vi "App - analyze RUS V6.vi"() -> ()   [LabVIEW 2015] (continued)
"phase"=4.207063834838992, "Q"=7083.997208863392, "Norm  Ampl"=0.042629920830408, "z (inf)"=0.4164640226070026-0.2153386241198867i, "4corners"={"z (-pi/2)"=-0.19933862411988668-0.3924640226070026i, "z(inf)"=0.4164640226070026-0.2153386241198867i, "z (pi/2)"=0.2393386241198867+0.4004640226070026i, "z center"=0.020000000000000018+0.0040000000000000036i, "z(0)"=-0.37646402260700257+0.2233386241198867i, "radius"=0.4530928748640071}}, "timestamp(min)"=241.9666666686535, "timestamp"=timestamp(3493742339 s since 1904-01-01), "Magn Field(T)"=0.0}, {"temperature"=175.963, "lorentzian"={"Amplitude"=0.0005260699966110523, "omega(0)"=666.5273905158227, "Gamma"=0.09447421907192355, "phase"=4.195778497264702, "Q"=7055.124636789992, "Norm  Ampl"=0.042809672171456516, "z (inf)"=0.41400103807529176-0.21982010606648514i, "4corners"={"z (-pi/2)"=-0.20382010606648512-0.39000103807529174i, "z(inf)"=0.41400103807529176-0.21982010606648514i, "z (pi/2)"=0.24382010606648516+0.39800103807529175i, "z center"=0.020000000000000018+0.0040000000000000036i, "z(0)"=-0.3740010380752917+0.22782010606648515i, "radius"=0.45313602580684326}}, "timestamp(min)"=243.2833333313465, "timestamp"=timestamp(3493742418 s since 1904-01-01), "Magn Field(T)"=0.0}, {"temperature"=175.634, "lorentzian"={"Amplitude"=0.000521344887977522, "omega(0)"=666.5408565163474, "Gamma"=0.09513732241648067, "phase"=4.19366498389086, "Q"=7006.092242100796, "Norm  Ampl"=0.04303036973253523, "z (inf)"=0.4127988612141764-0.22823659659492584i, "4corners"={"z (-pi/2)"=-0.20423659659492582-0.3967988612141764i, "z(inf)"=0.4127988612141764-0.22823659659492584i, "z (pi/2)"=0.24423659659492586+0.3887988612141764i, "z center"=0.020000000000000018-0.0040000000000000036i, "z(0)"=-0.3727988612141764+0.22023659659492584i, "radius"=0.4522974647548108}}, "timestamp(min)"=244.60000000149012, "timestamp"=timestamp(3493742497 s since 1904-01-01), "Magn Field(T)"=0.0}, {"temperature"=175.302, "lorentzian"={"Amplitude"=0.0005173979173400528, "omega(0)"=666.5638551761065, "Gamma"=0.0938468907422214, "phase"=4.179539778200027, "Q"=7102.6738329245645, "Norm  Ampl"=0.04236278976880251, "z (inf)"=0.40882213382141586-0.2333081460968691i, "4corners"={"z (-pi/2)"=-0.20930814609686907-0.39282213382141584i, "z(inf)"=0.40882213382141586-0.2333081460968691i, "z (pi/2)"=0.2493081460968691+0.38482213382141583i, "z center"=0.020000000000000018-0.0040000000000000036i, "z(0)"=-0.3688221338214158+0.22530814609686908i, "radius"=0.4514032317294839}}, "timestamp(min)"=245.93333333730698, "timestamp"=timestamp(3493742577 s since 1904-01-01), "Magn Field(T)"=0.0}, {"temperature"=174.985, "lorentzian"={"Amplitude"=0.0005254947174563582, "omega(0)"=666.584524931986, "Gamma"=0.09467228615844603, "phase"=4.174992240459032, "Q"=7040.967869059089, "Norm  Ampl"=0.04284549568400563, "z (inf)"=0.40877454210818925-0.22766937952883107i, "4corners"={"z (-pi/2)"=-0.21166937952883105-0.38477454210818923i, "z(inf)"=0.40877454210818925-0.22766937952883107i, "z (pi/2)"=0.25166937952883106+0.39277454210818924i, "z center"=0.020000000000000018+0.0040000000000000036i, "z(0)"=-0.3687745421081892+0.23566937952883107i, "radius"=0.4525663995511662}}, "timestamp(min)"=247.25, "timestamp"=timestamp(3493742656 s since 1904-01-01), "Magn Field(T)"=0.0}, {"temperature"=174.654, "lorentzian"={"Amplitude"=0.0005181490056271822, "omega(0)"=666.5994517164672, "Gamma"=0.09372303123313948, "phase"=4.158300486836943, "Q"=7112.440164875554, "Norm  Ampl"=0.042653947239770486, "z (inf)"=0.40701352496332366-0.2354625794994841i, "4corners"={"z (-pi/2)"=-0.21946257949948408-0.38301352496332364i, "z(inf)"=0.40701352496332366-0.2354625794994841i, "z (pi/2)"=0.25946257949948415+0.39101352496332364i, "z center"=0.020000000000000018+0.0040000000000000036i, "z(0)"=-0.3670135249633236+0.2434625794994841i, "radius"=0.4551063562345442}}, "timestamp(min)"=248.5666666701436, "timestamp"=timestamp(3493742735 s since 1904-01-01), "Magn Field(T)"=0.0}, {"temperature"=174.316, "lorentzian"={"Amplitude"=0.0005205950851143368, "omega(0)"=666.6209744644639, "Gamma"=0.09378760365181929, "phase"=4.155628442977468, "Q"=7107.772760025443, "Norm  Ampl"=0.04260755617709387, "z (inf)"=0.4056863388300806-0.23606887328625673i, "4corners"={"z (-pi/2)"=-0.2200688732862567-0.3816863388300806i, "z(inf)"=0.4056863388300806-0.23606887328625673i, "z (pi/2)"=0.2600688732862567+0.3896863388300806i, "z center"=0.020000000000000018+0.0040000000000000036i, "z(0)"=-0.36568633883008056+0.24406887328625673i, "radius"=0.4542983775901962}}, "timestamp(min)"=249.89999999850988, "timestamp"=timestamp(3493742815 s since 1904-01-01), "Magn Field(T)"=0.0}, {"temperature"=173.984, "lorentzian"={"Amplitude"=0.0005205939429529912, "omega(0)"=666.6398754592545, "Gamma"=0.09417963894260288, "phase"=4.150745972928352, "Q"=7078.386400117052, "Norm  Ampl"=0.04256979081159615, "z (inf)"=0.4025696519710433-0.23672840118410748i, "4corners"={"z (-pi/2)"=-0.22072840118410747-0.37856965197104325i, "z(inf)"=0.4025696519710433-0.23672840118410748i, "z (pi/2)"=0.2607284011841075+0.38656965197104326i, "z center"=0.020000000000000018+0.0040000000000000036i, "z(0)"=-0.36256965197104324+0.2447284011841075i, "radius"=0.4520063071970365}}, "timestamp(min)"=251.2166666686535, "timestamp"=timestamp(3493742894 s since 1904-01-01), "Magn Field(T)"=0.0}, {"temperature"=173.642, "lorentzian"={"Amplitude"=0.0005241695908499409, "omega(0)"=666.6584173096262, "Gamma"=0.09555208085544614, "phase"=4.155181311724554, "Q"=6976.91155798235, "Norm  Ampl"=0.04284869920904903, "z (inf)"=0.40060074366188225-0.24113954351394265i, "4corners"={"z (-pi/2)"=-0.21713954351394263-0.38460074366188224i, "z(inf)"=0.40060074366188225-0.24113954351394265i, "z (pi/2)"=0.25713954351394264+0.37660074366188223i, "z center"=0.020000000000000018-0.0040000000000000036i, "z(0)"=-0.3606007436618822+0.23313954351394264i, "radius"=0.44843292605915874}}, "timestamp(min)"=252.5333333313465, "timestamp"=timestamp(3493742973 s since 1904-01-01), "Magn Field(T)"=0.0}, {"temperature"=173.314, "lorentzian"={"Amplitude"=0.0005150928762822398, "omega(0)"=666.6738278296584, "Gamma"=0.09412889843388439, "phase"=4.129734532080279, "Q"=7082.562729637449, "Norm  Ampl"=0.04289883674194833, "z (inf)"=0.40054990465830365-0.24677056194440344i, "4corners"={"z (-pi/2)"=-0.23077056194440343-0.3765499046583036i, "z(inf)"=0.40054990465830365-0.24677056194440344i, "z (pi/2)"=0.27077056194440347+0.38454990465830363i, "z center"=0.020000000000000018+0.0040000000000000036i, "z(0)"=-0.3605499046583036+0.25477056194440345i, "radius"=0.45574565787657906}}, "timestamp(min)"=253.86666666716337, "timestamp"=timestamp(3493743053 s since 1904-01-01), "Magn Field(T)"=0.0}, {"temperature"=172.974, "lorentzian"={"Amplitude"=0.000516799692195644, "omega(0)"=666.692959166971, "Gamma"=0.09447287477688024, "phase"=4.135429912242744, "Q"=7056.977579453596, "Norm  Ampl"=0.042827204817983404, "z (inf)"=0.39994570670003854-0.24328038289100967i, "4corners"={"z (-pi/2)"=-0.22728038289100966-0.3759457067000385i, "z(inf)"=0.39994570670003854-0.24328038289100967i, "z (pi/2)"=0.2672803828910097+0.3839457067000385i, "z center"=0.020000000000000018+0.0040000000000000036i, "z(0)"=-0.3599457067000385+0.2512803828910097i, "radius"=0.4533280575946254}}, "timestamp(min)"=255.18333333730698, "timestamp"=timestamp(3493743132 s since 1904-01-01), "Magn Field(T)"=0.0}, {"temperature"=172.632, "lorentzian"={"Amplitude"=0.0005164262361548908, "omega(0)"=666.7084573649482, "Gamma"=0.09525334912451694, "phase"=4.119362082283542, "Q"=6999.3177509529305, "Norm  Ampl"=0.04303615866166019, "z (inf)"=0.3946624823159162-0.24850319278065613i, "4corners"={"z (-pi/2)"=-0.23250319278065612-0.3706624823159162i, "z(inf)"=0.3946624823159162-0.24850319278065613i, "z (pi/2)"=0.27250319278065616+0.3786624823159162i, "z center"=0.020000000000000018+0.0040000000000000036i, "z(0)"=-0.3546624823159162+0.25650319278065614i, "radius"=0.45180730186612683}}, "timestamp(min)"=256.5, "timestamp"=timestamp(3493743211 s since 1904-01-01), "Magn Field(T)"=0.0}, {"temperature"=172.303, "lorentzian"={"Amplitude"=0.0005144419777848418, "omega(0)"=666.7295180919369, "Gamma"=0.09498586850167676, "phase"=4.11250549518927, "Q"=7019.249585322972, "Norm  Ampl"=0.04256383601987101, "z (inf)"=0.3898681744046229-0.24897717189284335i, "4corners"={"z (-pi/2)"=-0.23297717189284334-0.3658681744046229i, "z(inf)"=0.3898681744046229-0.24897717189284335i, "z (pi/2)"=0.2729771718928434+0.3738681744046229i, "z center"=0.020000000000000018+0.0040000000000000036i, "z(0)"=-0.34986817440462287+0.25697717189284336i, "radius"=0.44810703624949894}}, "timestamp(min)"=257.83333333581686, "timestamp"=timestamp(3493743291 s since 1904-01-01), "Magn Field(T)"=0.0}, {"temperature"=171.947, "lorentzian"={"Amplitude"=0.0005056516743748706, "omega(0)"=666.7478022514588, "Gamma"=0.09481296917232077, "phase"=4.084832371198923, "Q"=7032.242614822634, "Norm  Ampl"=0.0422584021142444, "z (inf)"=0.38878060950325605-0.24970269914437565i, "4corners"={"z (-pi/2)"=-0.23370269914437564-0.348780609503256i, "z(inf)"=0.38878060950325605-0.24970269914437565i, "z (pi/2)"=0.2897026991443757+0.37278060950325603i, "z center"=0.028000000000000025+0.01200000000000001i, "z(0)"=-0.332780609503256+0.27370269914437567i, "radius"=0.44570276074194615}}, "timestamp(min)"=259.1499999985099, "timestamp"=timestamp(3493743370 s since 1904-01-01), "Magn Field(T)"=0.0}, {"temperature"=171.593, "lorentzian"={"Amplitude"=0.0004999937810113293, "omega(0)"=666.7684075589387, "Gamma"=0.07716584127533078, "phase"=4.101848615846865, "Q"=8640.71973478372, "Norm  Ampl"=0.04197129217223431, "z (inf)"=0.37764652347352495-0.2678293416658969i, "4corners"={"z (-pi/2)"=-0.37982934166589694-0.4016465234735249i, "z(inf)"=0.37764652347352495-0.2678293416658969i, "z (pi/2)"=0.24382934166589693+0.489646523473525i, "z center"=-0.068+0.04400000000000004i, "z(0)"=-0.513646523473525+0.35582934166589697i, "radius"=0.5439102519789691}}, "timestamp(min)"=260.4666666686535, "timestamp"=timestamp(3493743449 s since 1904-01-01), "Magn Field(T)"=0.0}, {"temperature"=171.216, "lorentzian"={"Amplitude"=0.0004971178519728986, "omega(0)"=666.7892001669214, "Gamma"=0.07709429273268266, "phase"=4.122089168704795, "Q"=8649.008591063302, "Norm  Ampl"=0.04142514157990056, "z (inf)"=0.37840040980273176-0.26308378893787776i, "4corners"={"z (-pi/2)"=-0.3670837889378778-0.41040040980273174i, "z(inf)"=0.37840040980273176-0.26308378893787776i, "z (pi/2)"=0.2310837889378778+0.4824004098027318i, "z center"=-0.068+0.03600000000000003i, "z(0)"=-0.5144004098027317+0.3350837889378778i, "radius"=0.5373308465717224}}, "timestamp(min)"=261.80000000447035, "timestamp"=timestamp(3493743529 s since 1904-01-01), "Magn Field(T)"=0.0}, {"temperature"=170.839, "lorentzian"={"Amplitude"=0.0005456618128673867, "omega(0)"=666.8168017277993, "Gamma"=0.10284084968364095, "phase"=4.2580332816999835, "Q"=6483.9682264300745, "Norm  Ampl"=0.0455123865470925, "z (inf)"=0.4016521142220204-0.26222859964929973i, "4corners"={"z (-pi/2)"=-0.19022859964929972-0.4656521142220204i, "z(inf)"=0.4016521142220204-0.26222859964929973i, "z (pi/2)"=0.19822859964929973+0.3296521142220204i, "z center"=0.0040000000000000036-0.068i, "z(0)"=-0.3936521142220204+0.12622859964929972i, "radius"=0.4425516386445436}}, "timestamp(min)"=263.1166666671634, "timestamp"=timestamp(3493743608 s since 1904-01-01), "Magn Field(T)"=0.0}, {"temperature"=170.496, "lorentzian"={"Amplitude"=0.0005526211872780759, "omega(0)"=666.8378173116613, "Gamma"=0.1050772709506424, "phase"=4.262296084777731, "Q"=6346.166124022129, "Norm  Ampl"=0.04629332333343278, "z (inf)"=0.40068729260806996-0.26766725748477393i, "4corners"={"z (-pi/2)"=-0.18766725748477392-0.47268729260806996i, "z(inf)"=0.40068729260806996-0.26766725748477393i, "z (pi/2)"=0.19566725748477393+0.32068729260806994i, "z center"=0.0040000000000000036-0.07600000000000001i, "z(0)"=-0.39268729260806995+0.11566725748477391i, "radius"=0.44056457609351113}}, "timestamp(min)"=264.45000000298023, "timestamp"=timestamp(3493743688 s since 1904-01-01), "Magn Field(T)"=0.0}, {"temperature"=170.187, "lorentzian"={"Amplitude"=0.0005512178829958511, "omega(0)"=666.8546119137043, "Gamma"=0.1059345471746253, "phase"=4.253770018900702, "Q"=6294.968258224992, "Norm  Ampl"=0.04649210092161766, "z (inf)"=0.40552439092601306-0.27029475928406893i, "4corners"={"z (-pi/2)"=-0.1822947592840689-0.46952439092601306i, "z(inf)"=0.40552439092601306-0.27029475928406893i, "z (pi/2)"=0.20629475928406893+0.31752439092601303i, "z center"=0.01200000000000001-0.07600000000000001i, "z(0)"=-0.38152439092601304+0.1182947592840689i, "radius"=0.43887572243055756}}, "timestamp(min)"=265.76666666567326, "timestamp"=timestamp(3493743767 s since 1904-01-01), "Magn Field(T)"=0.0}, {"temperature"=169.921, "lorentzian"={"Amplitude"=0.0004534509670476978, "omega(0)"=666.8518486216516, "Gamma"=0.07873324505819844, "phase"=3.841128173882247, "Q"=8469.762018937803, "Norm  Ampl"=0.03687627973060844, "z (inf)"=0.3295657315836148-0.3543691454307535i, "4corners"={"z (-pi/2)"=-0.33036914543075346-0.29756573158361477i, "z(inf)"=0.3295657315836148-0.3543691454307535i, "z (pi/2)"=0.3863691454307535+0.3055657315836148i, "z center"=0.028000000000000025+0.0040000000000000036i, "z(0)"=-0.27356573158361475+0.3623691454307535i, "radius"=0.46836986972085354}}, "timestamp(min)"=267.08333333581686, "timestamp"=timestamp(3493743846 s since 1904-01-01), "Magn Field(T)"=0.0}, {"temperature"=169.62, "lorentzian"={"Amplitude"=0.0004577554109132157, "omega(0)"=666.8670899449811, "Gamma"=0.07921421145205408, "phase"=3.886971896135157, "Q"=8418.52841454611, "Norm  Ampl"=0.037144170714167916, "z (inf)"=0.34603704562405213-0.340567947100091i, "4corners"={"z (-pi/2)"=-0.31656794710009095-0.3140370456240521i, "z(inf)"=0.34603704562405213-0.340567947100091i, "z (pi/2)"=0.372567947100091+0.3220370456240521i, "z center"=0.028000000000000025+0.0040000000000000036i, "z(0)"=-0.2900370456240521+0.348567947100091i, "radius"=0.4689079147956947}}, "timestamp(min)"=268.41666666418314, "timestamp"=timestamp(3493743926 s since 1904-01-01), "Magn Field(T)"=0.0}, {"temperature"=169.281, "lorentzian"={"Amplitude"=0.00046944630009999427, "omega(0)"=666.8864924413293, "Gamma"=0.08140026041873821, "phase"=3.8927509584525866, "Q"=8192.682541932176, "Norm  Ampl"=0.03810852720739882, "z (inf)"=0.3555140821106168-0.33817922533891204i, "4corners"={"z (-pi/2)"=-0.306179225338912-0.31551408211061677i, "z(inf)"=0.3555140821106168-0.33817922533891204i, "z (pi/2)"=0.3781792253389121+0.3235140821106168i, "z center"=0.03600000000000003+0.0040000000000000036i, "z(0)"=-0.28351408211061674+0.34617922533891204i, "radius"=0.46816222713983224}}, "timestamp(min)"=269.73333333432674, "timestamp"=timestamp(3493744005 s since 1904-01-01), "Magn Field(T)"=0.0}, {"temperature"=168.934, "lorentzian"={"Amplitude"=0.0004819119123264662, "omega(0)"=666.9049225640731, "Gamma"=0.08428016108055618, "phase"=3.9625507106763167, "Q"=7912.952633379947, "Norm  Ampl"=0.03935184782972083, "z (inf)"=0.3776895090479562-0.3142135310893408i, "4corners"={"z (-pi/2)"=-0.2822135310893408-0.33768950904795614i, "z(inf)"=0.3776895090479562-0.3142135310893408i, "z (pi/2)"=0.35421353108934084+0.34568950904795614i, "z center"=0.03600000000000003+0.0040000000000000036i, "z(0)"=-0.3056895090479561+0.3222135310893408i, "radius"=0.46691709324223735}}, "timestamp(min)"=271.05000000447035, "timestamp"=timestamp(3493744084 s since 1904-01-01), "Magn Field(T)"=0.0}, {"temperature"=168.567, "lorentzian"={"Amplitude"=0.00047042517655521463, "omega(0)"=666.9154225888688, "Gamma"=0.08165669931390285, "phase"=3.811505793800036, "Q"=8167.308110570664, "Norm  Ampl"=0.03849323915197239, "z (inf)"=0.32070276046478424-0.36552156103182776i, "4corners"={"z (-pi/2)"=-0.34152156103182774-0.2887027604647842i, "z(inf)"=0.32070276046478424-0.36552156103182776i, "z (pi/2)"=0.3975215610318278+0.2967027604647842i, "z center"=0.028000000000000025+0.0040000000000000036i, "z(0)"=-0.2647027604647842+0.37352156103182776i, "radius"=0.47140331994068907}}, "timestamp(min)"=272.3833333328366, "timestamp"=timestamp(3493744164 s since 1904-01-01), "Magn Field(T)"=0.0}, {"temperature"=168.198, "lorentzian"={"Amplitude"=0.0004781228250890849, "omega(0)"=666.9360592058572, "Gamma"=0.08225432815562943, "phase"=3.827463656766192, "Q"=8108.218426439273, "Norm  Ampl"=0.03910988481638956, "z (inf)"=0.3371408667391544-0.36395481797701695i, "4corners"={"z (-pi/2)"=-0.3319548179770169-0.29714086673915435i, "z(inf)"=0.3371408667391544-0.36395481797701695i, "z (pi/2)"=0.403954817977017+0.30514086673915436i, "z center"=0.03600000000000003+0.0040000000000000036i, "z(0)"=-0.2651408667391543+0.37195481797701696i, "radius"=0.4754750989199211}}, "timestamp(min)"=273.70000000298023, "timestamp"=timestamp(3493744243 s since 1904-01-01), "Magn Field(T)"=0.0}, {"temperature"=166.235, "lorentzian"={"Amplitude"=0.00047412858472916974, "omega(0)"=666.9893085918818, "Gamma"=0.08335043874440105, "phase"=3.9520200721143324, "Q"=8002.229126078666, "Norm  Ampl"=0.03905346852303167, "z (inf)"=0.37549950878743527-0.3189162721305466i, "4corners"={"z (-pi/2)"=-0.28691627213054655-0.33549950878743523i, "z(inf)"=0.37549950878743527-0.3189162721305466i, "z (pi/2)"=0.3589162721305466+0.34349950878743524i, "z center"=0.03600000000000003+0.0040000000000000036i, "z(0)"=-0.3034995087874352+0.3269162721305466i, "radius"=0.46854544632682005}}, "timestamp(min)"=275.01666666567326, "timestamp"=timestamp(3493744322 s since 1904-01-01), "Magn Field(T)"=0.0}, {"temperature"=167.465, "lorentzian"={"Amplitude"=0.00046785835178995565, "omega(0)"=667.023179450894, "Gamma"=0.08370886544636703, "phase"=4.015493047204771, "Q"=7968.3696092890095, "Norm  Ampl"=0.03886231878697336, "z (inf)"=0.39200901049802483-0.2939781015424444i, "4corners"={"z (-pi/2)"=-0.2619781015424444-0.3520090104980248i, "z(inf)"=0.39200901049802483-0.2939781015424444i, "z (pi/2)"=0.33397810154244445+0.3600090104980248i, "z center"=0.03600000000000003+0.0040000000000000036i, "z(0)"=-0.32000901049802477+0.3019781015424444i, "radius"=0.4642557103091162}}, "timestamp(min)"=276.3500000014901, "timestamp"=timestamp(3493744402 s since 1904-01-01), "Magn Field(T)"=0.0}, {"temperature"=167.68, "lorentzian"={"Amplitude"=0.0004660283199917108, "omega(0)"=667.0181290997397, "Gamma"=0.08122368655390495, "phase"=3.7880903220953956, "Q"=8212.11345359295, "Norm  Ampl"=0.03848331962891363, "z (inf)"=0.32141110368516546-0.37418188694120114i, "4corners"={"z (-pi/2)"=-0.3421818869412011-0.2814111036851654i, "z(inf)"=0.32141110368516546-0.37418188694120114i, "z (pi/2)"=0.41418188694120117+0.2894111036851654i, "z center"=0.03600000000000003+0.0040000000000000036i, "z(0)"=-0.2494111036851654+0.38218188694120114i, "radius"=0.4737942989496514}}, "timestamp(min)"=277.66666666418314, "timestamp"=timestamp(3493744481 s since 1904-01-01), "Magn Field(T)"=0.0}, {"temperature"=166.454, "lorentzian"={"Amplitude"=0.0004566778114597476, "omega(0)"=667.0522165263105, "Gamma"=0.07892871012914685, "phase"=3.8054289698611607, "Q"=8451.32544843123, "Norm  Ampl"=0.037899071353994104, "z (inf)"=0.33185238645268195-0.3741970972536763i, "4corners"={"z (-pi/2)"=-0.34219709725367625-0.2918523864526819i, "z(inf)"=0.33185238645268195-0.3741970972536763i, "z (pi/2)"=0.4141970972536763+0.2998523864526819i, "z center"=0.03600000000000003+0.0040000000000000036i, "z(0)"=-0.2598523864526819+0.3821970972536763i, "radius"=0.48016838602812423}}, "timestamp(min)"=279.0, "timestamp"=timestamp(3493744561 s since 1904-01-01), "Magn Field(T)"=0.0}, {"temperature"=166.595, "lorentzian"={"Amplitude"=0.0004415693097046763, "omega(0)"=667.0670953246381, "Gamma"=0.07763656776163326, "phase"=3.7695376107360197, "Q"=8592.176529141876, "Norm  Ampl"=0.036969393864618304, "z (inf)"=0.31575077270099183-0.3813465507477374i, "4corners"={"z (-pi/2)"=-0.34934655074773735-0.2757507727009918i, "z(inf)"=0.31575077270099183-0.3813465507477374i, "z (pi/2)"=0.4213465507477374+0.2837507727009918i, "z center"=0.03600000000000003+0.0040000000000000036i, "z(0)"=-0.24375077270099177+0.3893465507477374i, "radius"=0.47618532001730224}}, "timestamp(min)"=280.3166666701436, "timestamp"=timestamp(3493744640 s since 1904-01-01), "Magn Field(T)"=0.0}, {"temperature"=166.194, "lorentzian"={"Amplitude"=0.0004410364115785352, "omega(0)"=667.0830991408355, "Gamma"=0.07798823890009401, "phase"=3.736057416827716, "Q"=8553.637170796934, "Norm  Ampl"=0.03678081551395129, "z (inf)"=0.3001380691745166-0.37871285163862145i, "4corners"={"z (-pi/2)"=-0.35471285163862143-0.25213806917451653i, "z(inf)"=0.3001380691745166-0.37871285163862145i, "z (pi/2)"=0.4267128516386215+0.27613806917451655i, "z center"=0.03600000000000003+0.01200000000000001i, "z(0)"=-0.2281380691745165+0.40271285163862147i, "radius"=0.4716200292850433}}, "timestamp(min)"=281.6333333328366, "timestamp"=timestamp(3493744719 s since 1904-01-01), "Magn Field(T)"=0.0}, {"temperature"=165.738, "lorentzian"={"Amplitude"=0.0005310970253922922, "omega(0)"=667.0958987277553, "Gamma"=0.09231982716144078, "phase"=3.629992242151525, "Q"=7225.92230985438, "Norm  Ampl"=0.0441283586693555, "z (inf)"=0.3322812686918484-0.4421096316191092i, "4corners"={"z (-pi/2)"=-0.3141096316191092-0.2442812686918484i, "z(inf)"=0.3322812686918484-0.4421096316191092i, "z (pi/2)"=0.5301096316191092+0.20428126869184837i, "z center"=0.10799999999999998-0.020000000000000018i, "z(0)"=-0.1162812686918484+0.4021096316191092i, "radius"=0.4779943813389914}}, "timestamp(min)"=282.9666666686535, "timestamp"=timestamp(3493744799 s since 1904-01-01), "Magn Field(T)"=0.0}, {"temperature"=165.506, "lorentzian"={"Amplitude"=0.0004453500100210904, "omega(0)"=667.1178151875246, "Gamma"=0.07879774106191258, "phase"=3.724253916429, "Q"=8466.204820051376, "Norm  Ampl"=0.03683544160772606, "z (inf)"=0.29322348499012246-0.386336569477198i, "4corners"={"z (-pi/2)"=-0.354336569477198-0.2532234849901224i, "z(inf)"=0.29322348499012246-0.386336569477198i, "z (pi/2)"=0.42633656947719806+0.26122348499012243i, "z center"=0.03600000000000003+0.0040000000000000036i, "z(0)"=-0.2212234849901224+0.39433656947719803i, "radius"=0.46746824352215754}}, "timestamp(min)"=284.2833333313465, "timestamp"=timestamp(3493744878 s since 1904-01-01), "Magn Field(T)"=0.0}, {"temperature"=165.119, "lorentzian"={"Amplitude"=0.0005157776397258885, "omega(0)"=667.1376282461717, "Gamma"=0.09116435635561218, "phase"=3.709814210705731, "Q"=7317.965649247981, "Norm  Ampl"=0.04244970024471032, "z (inf)"=0.3585762630295389-0.41246837363300054i, "4corners"={"z (-pi/2)"=-0.28446837363300054-0.2705762630295389i, "z(inf)"=0.3585762630295389-0.41246837363300054i, "z (pi/2)"=0.5004683736330005+0.23057626302953887i, "z center"=0.10799999999999998-0.020000000000000018i, "z(0)"=-0.1425762630295389+0.3724683736330005i, "radius"=0.46563922504013894}}, "timestamp(min)"=285.6000000014901, "timestamp"=timestamp(3493744957 s since 1904-01-01), "Magn Field(T)"=0.0}, {"temperature"=164.781, "lorentzian"={"Amplitude"=0.0004418438472308204, "omega(0)"=667.1555761001051, "Gamma"=0.07827432143846805, "phase"=3.7454834472622567, "Q"=8523.300666675987, "Norm  Ampl"=0.03688829185154937, "z (inf)"=0.30361004228281907-0.3839171365651249i, "4corners"={"z (-pi/2)"=-0.35191713656512486-0.26361004228281903i, "z(inf)"=0.30361004228281907-0.3839171365651249i, "z (pi/2)"=0.4239171365651249+0.27161004228281904i, "z center"=0.03600000000000003+0.0040000000000000036i, "z(0)"=-0.231610042282819+0.3919171365651249i, "radius"=0.4712693917193201}}, "timestamp(min)"=286.933333337307, "timestamp"=timestamp(3493745037 s since 1904-01-01), "Magn Field(T)"=0.0}, {"temperature"=164.449, "lorentzian"={"Amplitude"=0.00043959014352216384, "omega(0)"=667.1729816030107, "Gamma"=0.07792122289310302, "phase"=3.7572404166451623, "Q"=8562.147215249412, "Norm  Ampl"=0.03705674417312184, "z (inf)"=0.31063385325452725-0.3842524925874322i, "4corners"={"z (-pi/2)"=-0.3522524925874322-0.2706338532545272i, "z(inf)"=0.31063385325452725-0.3842524925874322i, "z (pi/2)"=0.42425249258743225+0.2786338532545272i, "z center"=0.03600000000000003+0.0040000000000000036i, "z(0)"=-0.23863385325452718+0.3922524925874322i, "radius"=0.4755667685549352}}, "timestamp(min)"=288.25, "timestamp"=timestamp(3493745116 s since 1904-01-01), "Magn Field(T)"=0.0}, {"temperature"=164.092, "lorentzian"={"Amplitude"=0.00044484134846526204, "omega(0)"=667.1877067469779, "Gamma"=0.07911173500148858, "phase"=3.73486561224118, "Q"=8433.485964306357, "Norm  Ampl"=0.037600025703834174, "z (inf)"=0.3017170249130602-0.382059819707589i, "4corners"={"z (-pi/2)"=-0.358059819707589-0.25371702491306014i, "z(inf)"=0.3017170249130602-0.382059819707589i, "z (pi/2)"=0.43005981970758905+0.27771702491306016i, "z center"=0.03600000000000003+0.01200000000000001i, "z(0)"=-0.22971702491306012+0.40605981970758903i, "radius"=0.4752774756251609}}, "timestamp(min)"=289.58333333581686, "timestamp"=timestamp(3493745196 s since 1904-01-01), "Magn Field(T)"=0.0}, {"temperature"=163.762, "lorentzian"={"Amplitude"=0.00042567935379481, "omega(0)"=667.2026820856647, "Gamma"=0.07477989988062614, "phase"=3.664321115162137, "Q"=8922.219515548222, "Norm  Ampl"=0.035311410368920784, "z (inf)"=0.27174628774594833-0.40514648048645424i, "4corners"={"z (-pi/2)"=-0.3731464804864542-0.23174628774594827i, "z(inf)"=0.27174628774594833-0.40514648048645424i, "z (pi/2)"=0.4451464804864543+0.23974628774594828i, "z center"=0.03600000000000003+0.0040000000000000036i, "z(0)"=-0.19974628774594824+0.41314648048645425i, "radius"=0.47220456867807614}}, "timestamp(min)"=290.8999999985099, "timestamp"=timestamp(3493745275 s since 1904-01-01), "Magn Field(T)"=0.0}, {"temperature"=163.413, "lorentzian"={"Amplitude"=0.00041595713785414265, "omega(0)"=667.2204079387552, "Gamma"=0.07270858758415784, "phase"=3.6652170850341648, "Q"=9176.638277651442, "Norm  Ampl"=0.0343363115045469, "z (inf)"=0.2641332990001735-0.40497063950565165i, "4corners"={"z (-pi/2)"=-0.38097063950565163-0.2321332990001735i, "z(inf)"=0.2641332990001735-0.40497063950565165i, "z (pi/2)"=0.4369706395056517+0.2401332990001735i, "z center"=0.028000000000000025+0.0040000000000000036i, "z(0)"=-0.20813329900017347+0.41297063950565166i, "radius"=0.47224561286937017}}, "timestamp(min)"=292.2166666686535, "timestamp"=timestamp(3493745354 s since 1904-01-01), "Magn Field(T)"=0.0}, {"temperature"=163.066, "lorentzian"={"Amplitude"=0.000412780965095534, "omega(0)"=667.2371268200717, "Gamma"=0.072148551218395, "phase"=3.6596651214491858, "Q"=9248.101528751875, "Norm  Ampl"=0.03428932453282723, "z (inf)"=0.26335185326350824-0.40089420742790194i, "4corners"={"z (-pi/2)"=-0.3848942074279019-0.2233518532635082i, "z(inf)"=0.26335185326350824-0.40089420742790194i, "z (pi/2)"=0.440894207427902+0.24735185326350823i, "z center"=0.028000000000000025+0.01200000000000001i, "z(0)"=-0.2073518532635082+0.42489420742790196i, "radius"=0.47526005656070364}}, "timestamp(min)"=293.55000000447035, "timestamp"=timestamp(3493745434 s since 1904-01-01), "Magn Field(T)"=0.0}, {"temperature"=162.731, "lorentzian"={"Amplitude"=0.0004102842033046791, "omega(0)"=667.2364415496808, "Gamma"=0.07209084985268063, "phase"=3.6064865792014325, "Q"=9255.4941842577, "Norm  Ampl"=0.033756126499018595, "z (inf)"=0.24592700578322318-0.4145490860197161i, "4corners"={"z (-pi/2)"=-0.38254908601971604-0.20592700578322315i, "z(inf)"=0.24592700578322318-0.4145490860197161i, "z (pi/2)"=0.4545490860197161+0.21392700578322316i, "z center"=0.03600000000000003+0.0040000000000000036i, "z(0)"=-0.17392700578322312+0.4225490860197161i, "radius"=0.46824425801610114}}, "timestamp(min)"=294.8666666671634, "timestamp"=timestamp(3493745513 s since 1904-01-01), "Magn Field(T)"=0.0}, {"temperature"=162.385, "lorentzian"={"Amplitude"=0.0003956527969362258, "omega(0)"=667.2762898680271, "Gamma"=0.06962769430773084, "phase"=3.717337149894252, "Q"=9583.48968039774, "Norm  Ampl"=0.03259572680926661, "z (inf)"=0.29088493539914-0.3806724598159571i, "4corners"={"z (-pi/2)"=-0.3566724598159571-0.24288493539913997i, "z(inf)"=0.29088493539914-0.3806724598159571i, "z (pi/2)"=0.42867245981595714+0.26688493539914i, "z center"=0.03600000000000003+0.01200000000000001i, "z(0)"=-0.21888493539913995+0.4046724598159571i, "radius"=0.4681431308812917}}, "timestamp(min)"=296.20000000298023, "timestamp"=timestamp(3493745593 s since 1904-01-01), "Magn Field(T)"=0.0}, {"temperature"=162.052, "lorentzian"={"Amplitude"=0.0003908194038920824, "omega(0)"=667.2972094216088, "Gamma"=0.060554526875683225, "phase"=3.818969248519727, "Q"=11019.774141602189, "Norm  Ampl"=0.032463602340691455, "z (inf)"=0.2840045144273522-0.3737437622419629i, "4corners"={"z (-pi/2)"=-0.4697437622419629-0.29200451442735215i, "z(inf)"=0.2840045144273522-0.3737437622419629i, "z (pi/2)"=0.3657437622419629+0.3800045144273522i, "z center"=-0.05199999999999999+0.04400000000000004i, "z(0)"=-0.3880045144273522+0.46174376224196295i, "radius"=0.5361052924637383}}, "timestamp(min)"=297.51666666567326, "timestamp"=timestamp(3493745672 s since 1904-01-01), "Magn Field(T)"=0.0}, {"temperature"=161.701, "lorentzian"={"Amplitude"=0.0004023371306905148, "omega(0)"=667.3167356990505, "Gamma"=0.07125599300957257, "phase"=3.771737078401076, "Q"=9365.06120417693, "Norm  Ampl"=0.03371176902153503, "z (inf)"=0.31478421296215664-0.37824389067415964i, "4corners"={"z (-pi/2)"=-0.3462438906741596-0.2747842129621566i, "z(inf)"=0.31478421296215664-0.37824389067415964i, "z (pi/2)"=0.4182438906741597+0.2827842129621566i, "z center"=0.03600000000000003+0.0040000000000000036i, "z(0)"=-0.24278421296215658+0.38624389067415965i, "radius"=0.47310784114686577}}, "timestamp(min)"=298.83333333581686, "timestamp"=timestamp(3493745751 s since 1904-01-01), "Magn Field(T)"=0.0}, {"temperature"=161.356, "lorentzian"={"Amplitude"=0.0003980448176269801, "omega(0)"=667.3324754640709, "Gamma"=0.07037664438589454, "phase"=3.7386617857270874, "Q"=9482.30028992151, "Norm  Ampl"=0.03310262150486229, "z (inf)"=0.3004484190328178-0.3769846776897172i, "4corners"={"z (-pi/2)"=-0.3529846776897172-0.2524484190328178i, "z(inf)"=0.3004484190328178-0.3769846776897172i, "z (pi/2)"=0.42498467768971726+0.2764484190328178i, "z center"=0.03600000000000003+0.01200000000000001i, "z(0)"=-0.22844841903281776+0.40098467768971724i, "radius"=0.4703637377671986}}, "timestamp(min)"=300.16666666418314, "timestamp"=timestamp(3493745831 s since 1904-01-01), "Magn Field(T)"=0.0}, {"temperature"=161.021, "lorentzian"={"Amplitude"=0.00040196216116563467, "omega(0)"=667.3490257970444, "Gamma"=0.07077241015125915, "phase"=3.7097897167890186, "Q"=9429.508255699431, "Norm  Ampl"=0.03329650708290407, "z (inf)"=0.2891677604628733-0.38454875486892365i, "4corners"={"z (-pi/2)"=-0.3605487548689236-0.24116776046287325i, "z(inf)"=0.2891677604628733-0.38454875486892365i, "z (pi/2)"=0.4325487548689237+0.26516776046287327i, "z center"=0.03600000000000003+0.01200000000000001i, "z(0)"=-0.21716776046287323+0.40854875486892367i, "radius"=0.4704729853305931}}, "timestamp(min)"=301.48333333432674, "timestamp"=timestamp(3493745910 s since 1904-01-01), "Magn Field(T)"=0.0}, {"temperature"=160.674, "lorentzian"={"Amplitude"=0.0004054841053044689, "omega(0)"=667.3649515647236, "Gamma"=0.07158288458859594, "phase"=3.690228810756028, "Q"=9322.968128488123, "Norm  Ampl"=0.03418277410279088, "z (inf)"=0.2850419090554205-0.4034436767226396i, "4corners"={"z (-pi/2)"=-0.37144367672263956-0.24504190905542042i, "z(inf)"=0.2850419090554205-0.4034436767226396i, "z (pi/2)"=0.4434436767226396+0.25304190905542046i, "z center"=0.03600000000000003+0.0040000000000000036i, "z(0)"=-0.2130419090554204+0.4114436767226396i, "radius"=0.4775271952122006}}, "timestamp(min)"=302.80000000447035, "timestamp"=timestamp(3493745989 s since 1904-01-01), "Magn Field(T)"=0.0}, {"temperature"=160.342, "lorentzian"={"Amplitude"=0.0003969949690495204, "omega(0)"=667.3831987020516, "Gamma"=0.06994734920807832, "phase"=3.6639418047607673, "Q"=9541.22216578544, "Norm  Ampl"=0.03306473488500743, "z (inf)"=0.2718426996797837-0.3976729553227081i, "4corners"={"z (-pi/2)"=-0.37367295532270806-0.22384269967978368i, "z(inf)"=0.2718426996797837-0.3976729553227081i, "z (pi/2)"=0.4456729553227081+0.2478426996797837i, "z center"=0.03600000000000003+0.01200000000000001i, "z(0)"=-0.19984269967978366+0.4216729553227081i, "radius"=0.47270890547470146}}, "timestamp(min)"=304.1333333328366, "timestamp"=timestamp(3493746069 s since 1904-01-01), "Magn Field(T)"=0.0}, {"temperature"=159.993, "lorentzian"={"Amplitude"=0.00040776573484213136, "omega(0)"=667.3988052282629, "Gamma"=0.07174331319710288, "phase"=3.6502540542629744, "Q"=9302.592471505952, "Norm  Ampl"=0.03398554650608507, "z (inf)"=0.2667009691273185-0.40973725036355885i, "4corners"={"z (-pi/2)"=-0.3777372503635588-0.22670096912731846i, "z(inf)"=0.2667009691273185-0.40973725036355885i, "z (pi/2)"=0.4497372503635589+0.23470096912731847i, "z center"=0.03600000000000003+0.0040000000000000036i, "z(0)"=-0.19470096912731844+0.41773725036355885i, "radius"=0.47371030123344593}}, "timestamp(min)"=305.45000000298023, "timestamp"=timestamp(3493746148 s since 1904-01-01), "Magn Field(T)"=0.0}, {"temperature"=159.648, "lorentzian"={"Amplitude"=0.0004680176889170384, "omega(0)"=667.4131682428546, "Gamma"=0.0812921215811641, "phase"=3.612504259131583, "Q"=8210.05966213457, "Norm  Ampl"=0.03863268738088678, "z (inf)"=0.3236126044639621-0.45150616925067943i, "4corners"={"z (-pi/2)"=-0.3155061692506794-0.24361260446396216i, "z(inf)"=0.3236126044639621-0.45150616925067943i, "z (pi/2)"=0.5315061692506794+0.1876126044639621i, "z center"=0.10799999999999998-0.028000000000000025i, "z(0)"=-0.10761260446396215+0.3955061692506794i, "radius"=0.47523285934067955}}, "timestamp(min)"=306.7833333313465, "timestamp"=timestamp(3493746228 s since 1904-01-01), "Magn Field(T)"=0.0}, {"temperature"=159.311, "lorentzian"={"Amplitude"=0.00039915939373379985, "omega(0)"=667.4308567999159, "Gamma"=0.07054690221192932, "phase"=3.624092222923141, "Q"=9460.810267683943, "Norm  Ampl"=0.033325757837266635, "z (inf)"=0.25518722235474023-0.40646230729603344i, "4corners"={"z (-pi/2)"=-0.3824623072960334-0.2071872223547402i, "z(inf)"=0.25518722235474023-0.40646230729603344i, "z (pi/2)"=0.4544623072960335+0.23118722235474023i, "z center"=0.03600000000000003+0.01200000000000001i, "z(0)"=-0.1831872223547402+0.43046230729603346i, "radius"=0.4723915124884297}}, "timestamp(min)"=308.1000000014901, "timestamp"=timestamp(3493746307 s since 1904-01-01), "Magn Field(T)"=0.0}, {"temperature"=158.97, "lorentzian"={"Amplitude"=0.0004048868300764196, "omega(0)"=667.4487531200956, "Gamma"=0.07079873108028, "phase"=3.6399859889647472, "Q"=9427.411239380308, "Norm  Ampl"=0.03364557728117188, "z (inf)"=0.2631663396406196-0.4134177943208631i, "4corners"={"z (-pi/2)"=-0.3814177943208631-0.22316633964061955i, "z(inf)"=0.2631663396406196-0.4134177943208631i, "z (pi/2)"=0.45341779432086315+0.23116633964061956i, "z center"=0.03600000000000003+0.0040000000000000036i, "z(0)"=-0.19116633964061952+0.4214177943208631i, "radius"=0.47522853542418064}}, "timestamp(min)"=309.41666666418314, "timestamp"=timestamp(3493746386 s since 1904-01-01), "Magn Field(T)"=0.0}, {"temperature"=158.635, "lorentzian"={"Amplitude"=0.00044686446108478477, "omega(0)"=667.4658300241209, "Gamma"=0.08063717245044377, "phase"=3.6566788015994365, "Q"=8277.396264536897, "Norm  Ampl"=0.03731426534314974, "z (inf)"=0.32795161363052017-0.43070199439036766i, "4corners"={"z (-pi/2)"=-0.30270199439036766-0.2559516136305202i, "z(inf)"=0.32795161363052017-0.43070199439036766i, "z (pi/2)"=0.5027019943903677+0.19995161363052016i, "z center"=0.09999999999999998-0.028000000000000025i, "z(0)"=-0.1279516136305202+0.3747019943903676i, "radius"=0.46274273029701685}}, "timestamp(min)"=310.75, "timestamp"=timestamp(3493746466 s since 1904-01-01), "Magn Field(T)"=0.0}, {"temperature"=158.293, "lorentzian"={"Amplitude"=0.0004385033400474334, "omega(0)"=667.4848884179092, "Gamma"=0.08087380716911047, "phase"=3.671755223868203, "Q"=8253.412467922659, "Norm  Ampl"=0.0364652352730877, "z (inf)"=0.3360034474521866-0.41699449182348824i, "4corners"={"z (-pi/2)"=-0.28099449182348823-0.2560034474521866i, "z(inf)"=0.3360034474521866-0.41699449182348824i, "z (pi/2)"=0.4969944918234882+0.20000344745218657i, "z center"=0.10799999999999998-0.028000000000000025i, "z(0)"=-0.1200034474521866+0.3609944918234882i, "radius"=0.45089054849164434}}, "timestamp(min)"=312.0666666701436, "timestamp"=timestamp(3493746545 s since 1904-01-01), "Magn Field(T)"=0.0}, {"temperature"=157.95, "lorentzian"={"Amplitude"=0.0003817963882074518, "omega(0)"=667.5023892207363, "Gamma"=0.06795073544754765, "phase"=3.66569095513469, "Q"=9823.328398498246, "Norm  Ampl"=0.03195987851025704, "z (inf)"=0.27137292227921667-0.39520796710072414i, "4corners"={"z (-pi/2)"=-0.3712079671007241-0.22337292227921662i, "z(inf)"=0.27137292227921667-0.39520796710072414i, "z (pi/2)"=0.4432079671007242+0.24737292227921664i, "z center"=0.03600000000000003+0.01200000000000001i, "z(0)"=-0.1993729222792166+0.41920796710072417i, "radius"=0.4703389639531926}}, "timestamp(min)"=313.3833333328366, "timestamp"=timestamp(3493746624 s since 1904-01-01), "Magn Field(T)"=0.0}, {"temperature"=157.609, "lorentzian"={"Amplitude"=0.00038130536815095435, "omega(0)"=667.5167865078748, "Gamma"=0.0677240559576261, "phase"=3.6387070758342603, "Q"=9856.420692309537, "Norm  Ampl"=0.031958127035959974, "z (inf)"=0.2610389431826826-0.40277122534397447i, "4corners"={"z (-pi/2)"=-0.37877122534397445-0.21303894318268254i, "z(inf)"=0.2610389431826826-0.40277122534397447i, "z (pi/2)"=0.4507712253439745+0.23703894318268257i, "z center"=0.03600000000000003+0.01200000000000001i, "z(0)"=-0.18903894318268252+0.4267712253439745i, "radius"=0.47188737567572275}}, "timestamp(min)"=314.7166666686535, "timestamp"=timestamp(3493746704 s since 1904-01-01), "Magn Field(T)"=0.0}, {"temperature"=157.261, "lorentzian"={"Amplitude"=0.00038861997515745363, "omega(0)"=667.530667219577, "Gamma"=0.06900808152994153, "phase"=3.6253379721641847, "Q"=9673.224532838894, "Norm  Ampl"=0.032631212191482246, "z (inf)"=0.2559265859576157-0.41460431438121875i, "4corners"={"z (-pi/2)"=-0.3826043143812187-0.21592658595761566i, "z(inf)"=0.2559265859576157-0.41460431438121875i, "z (pi/2)"=0.4546043143812188+0.22392658595761566i, "z center"=0.03600000000000003+0.0040000000000000036i, "z(0)"=-0.18392658595761563+0.42260431438121876i, "radius"=0.472860735554923}}, "timestamp(min)"=316.0333333313465, "timestamp"=timestamp(3493746783 s since 1904-01-01), "Magn Field(T)"=0.0}, {"temperature"=156.94, "lorentzian"={"Amplitude"=0.00043319241384855855, "omega(0)"=667.5446936387285, "Gamma"=0.0777817292430267, "phase"=3.589005980517976, "Q"=8582.281470665237, "Norm  Ampl"=0.036487522044557734, "z (inf)"=0.3109496683648186-0.45092742094241833i, "4corners"={"z (-pi/2)"=-0.3149274209424183-0.23094966836481862i, "z(inf)"=0.3109496683648186-0.45092742094241833i, "z (pi/2)"=0.5309274209424183+0.17494966836481857i, "z center"=0.10799999999999998-0.028000000000000025i, "z(0)"=-0.0949496683648186+0.3949274209424183i, "radius"=0.4691014509404073}}, "timestamp(min)"=317.3666666671634, "timestamp"=timestamp(3493746863 s since 1904-01-01), "Magn Field(T)"=0.0}, {"temperature"=156.59, "lorentzian"={"Amplitude"=0.00036686354960487164, "omega(0)"=667.5507361439306, "Gamma"=0.06764669851983329, "phase"=3.587535413817995, "Q"=9868.193877166257, "Norm  Ampl"=0.031896054674531896, "z (inf)"=0.23936607820909092-0.4213978828159163i, "4corners"={"z (-pi/2)"=-0.38939788281591625-0.19936607820909089i, "z(inf)"=0.23936607820909092-0.4213978828159163i, "z (pi/2)"=0.4613978828159163+0.2073660782090909i, "z center"=0.03600000000000003+0.0040000000000000036i, "z(0)"=-0.16736607820909086+0.4293978828159163i, "radius"=0.4715094065555958}}, "timestamp(min)"=318.683333337307, "timestamp"=timestamp(3493746942 s since 
